vi "Post-Install Custom Action.vi"() -> (0 "error out":errorcluster)   [LabVIEW 2021]
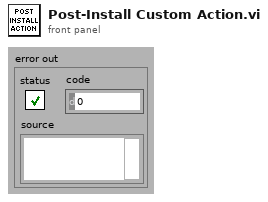
[diagram p1: front panel]
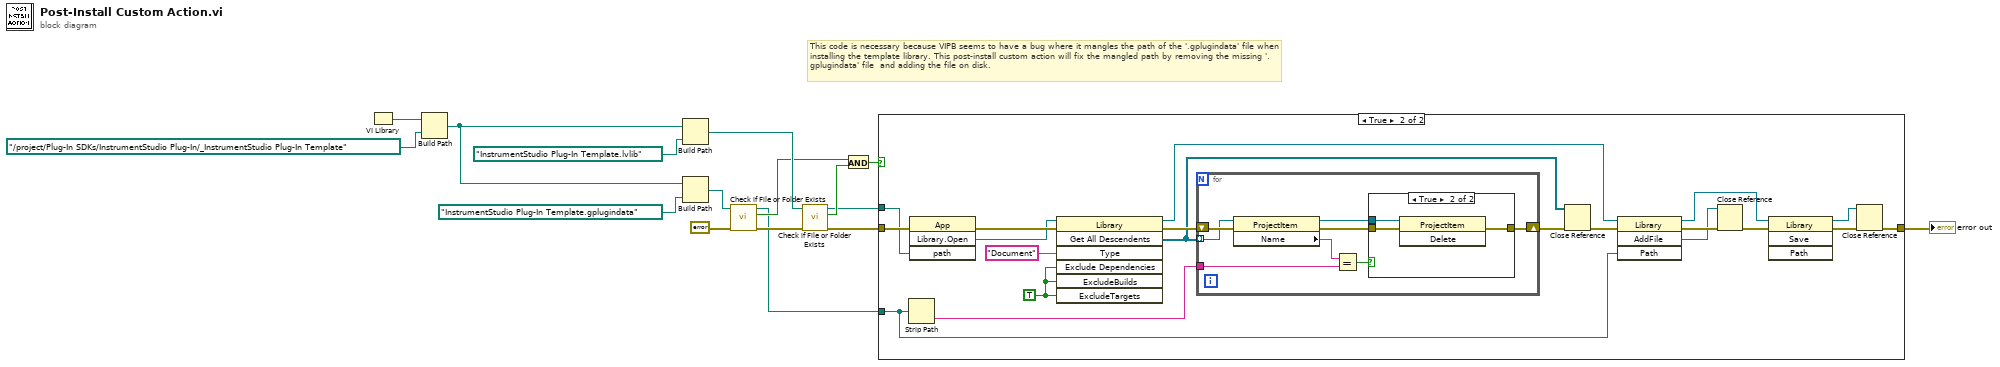
[diagram p0: block diagram]
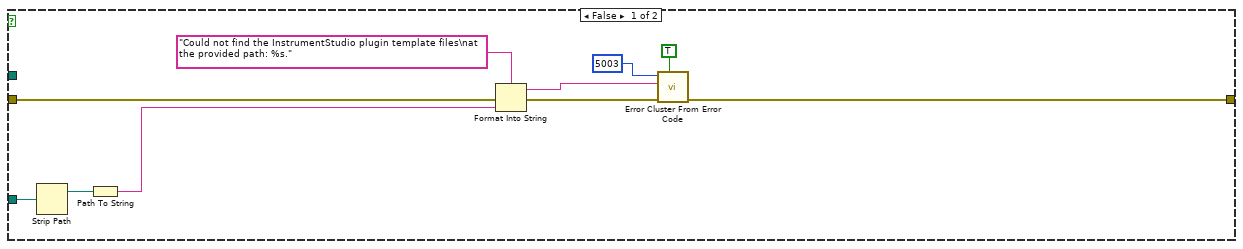
[diagram p2: hidden frame]
diagram:
  # "This code is necessary because VIPB seems to have a bug where it mangles the path of the '.gplugindata' file when installing the template library. This post-install custom action will fix the mangled path by removing the missing '.gplugindata' file  and adding the file on disk."
  n1 = VI Library() -> (path=w3:path)
  n2 = Build Path(base path=w3, name or relative path=path "../project/Plug-In SDKs/InstrumentStudio Plug-In/_InstrumentStudio Plug-In Template") -> (appended path=w1:path)
  n3 = Build Path(base path=w1, name or relative path=path "InstrumentStudio Plug-In Template.lvlib") -> (appended path=w14:path)
  n4 = Build Path(base path=w1, name or relative path=path "InstrumentStudio Plug-In Template.gplugindata") -> (appended path=w16:path)
  n5 = call <vilib>:"Check if File or Folder Exists.vi"("error in (no error)"=errorcluster {"status"=FALSE, "code"=0, "source"=""}, "path"=w16) -> ("error out"=w15:errorcluster, "file or folder exists?"=w13:bool, "dup path"=w7:path)  [unwired: 7 in]
  n6 = call <vilib>:"Check if File or Folder Exists.vi"("error in (no error)"=w15, "path"=w14) -> ("error out"=w10:errorcluster, "file or folder exists?"=w12:bool, "dup path"=w8:path)  [unwired: 7 in]
  n7 = And(x=w13, y=w12) -> (x .and. y?=w11:bool)
  n8 = case shown="True" w11 {
    tunnel: w10 -> [w26 w46]
    tunnel: [w25 w28] -> w6
    tunnel: w8 -> [_ w44]
    tunnel: w7 -> [w21 w33]
    frame False {
      n9 = Strip Path(path=w21) -> (stripped path=w20:path)  [unwired: 1 out]
      n10 = Path To String(path=w20) -> (string=w22:string)
      n11 = Format Into String(format string="Could not find the InstrumentStudio plugin template files\nat the provided path: %s." ("error message (\"\")"), error in=w26, w22) -> (resulting string=w18:string, error out=w23:errorcluster)  [unwired: 1 in]
      n12 = call <vilib>:"Error Cluster From Error Code.vi"("show call chain? (False)"=TRUE, "error in (no error)"=w23, "error message (\"\")"=w18, "error code (0)"=5003) -> ("error out"=w25:errorcluster)  [unwired: 5 in]
    }
    frame True {
      w41 = TRUE ("ExcludeTargets")
      n13 = Strip Path(path=w33) -> (name=w39:string)  [unwired: 1 out]
      n14 = invoke class="App" method="Library.Open"(error in=w46, "path"=w44) -> (error out=w45:errorcluster, "Open Library"=w43:refnum<vi>)  [unwired: 2 in, 2 out]
      n15 = invoke class="Library" method="Get All Descendents"(reference=w43, error in=w45, "Type"="Document", "Exclude Dependencies"=w41, "ExcludeBuilds"=w41, "ExcludeTargets"=w41) -> (reference out=w34:refnum<vi>, error out=w40:errorcluster, "All Descendents"=w36:refnum<vi>[])  [unwired: 1 in, 4 out]
      n16 = for {
        shift-right: [w49] -> w38
        shift-left: w40 -> [w54]
        tunnel: w36 -> [w53] mode=indexing
        tunnel: w39 -> [w51]
        n17 = property class="ProjectItem"(reference=w53, error in=w54) -> (reference out=w48:refnum<vi>, error out=w50:errorcluster, "Name"=w52:string)
        n18 = Equal?(x=w52, y=w51) -> (x = y?=w47:bool)
        n19 = case shown="True" w47 {
          tunnel: w50 -> [w55 w58]
          tunnel: [w55 w57] -> w49
          tunnel: w48 -> [_ w56]
          frame False {
          }
          frame True {
            n20 = invoke class="ProjectItem" method="Delete"(reference=w56, error in=w58) -> (error out=w57:errorcluster)  [unwired: 1 in, 2 out]
          }
        }
      }
      n21 = Close Reference(reference=w36, error in (no error)=w38) -> (error out=w37:errorcluster)
      n22 = invoke class="Library" method="AddFile"(reference=w34, error in=w37, "Path"=w33) -> (reference out=w29:refnum<vi>, error out=w35:errorcluster, "AddFile"=w30:refnum<vi>)  [unwired: 1 in, 1 out]
      n23 = Close Reference(reference=w30, error in (no error)=w35) -> (error out=w32:errorcluster)
      n24 = invoke class="Library" method="Save"(reference=w29, error in=w32) -> (reference out=w27:refnum<vi>, error out=w31:errorcluster)  [unwired: 2 in, 2 out]
      n25 = Close Reference(reference=w27, error in (no error)=w31) -> (error out=w28:errorcluster)
    }
  }
  "error out" <- w6
